vi "getRowElements.vi"(8 "error in (no error)":errorcluster, 11 "Category in":refnum<class "Category.lvclass">) -> (0 "error out":errorcluster, 2 "Row Interface":string[](array[string]), 3 "Category out":refnum<class "Category.lvclass">)   [LabVIEW 2020, in "Category.lvclass"]
uses:
  Category.lvclass
  UserEditableAmount/UserEditableAmount.lvclass
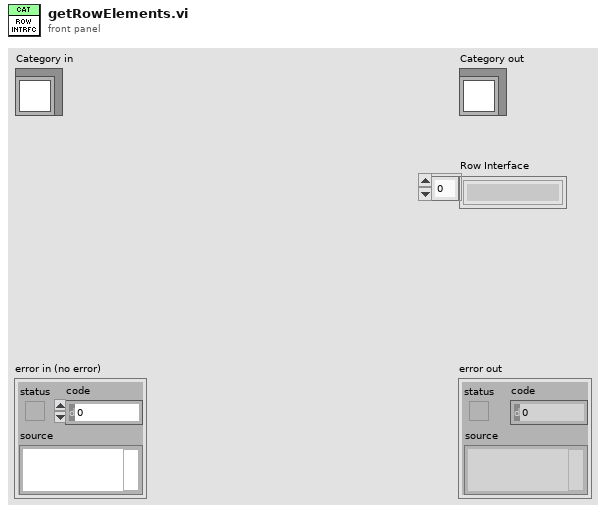
[diagram p1: front panel]
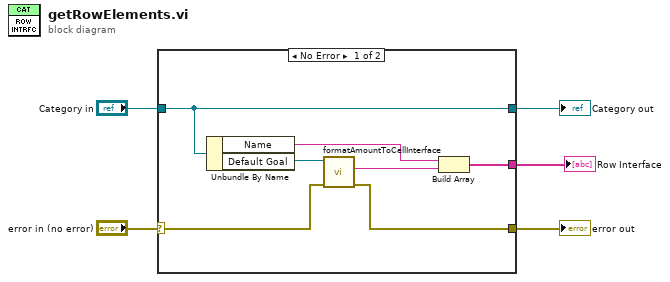
[diagram p0: block diagram]
diagram:
  n1 = case shown="No Error" "error in (no error)" {
    selector: "error in (no error)" -> [w12 w14]
    tunnel: [w11 w14] -> w4
    tunnel: [w7 w13] -> w2
    tunnel: "Category in" -> [w7 w13]
    tunnel: [w8 _] -> w1
    frame No Error {
      n2 = Unbundle By Name(w7) -> ("Name"=w10:string, "Default Goal"=w6:refnum<class "UserEditableAmount.lvclass">)
      n3 = call "formatAmountToCellInterface.vi"("error in (no error)"=w12, "UserEditableAmount in"=w6) -> ("error out"=w11:errorcluster, "Cell Interface"=w9:string)  [unwired: 7 in, 1 out]
      n4 = Build Array(w10, w9) -> (w8:string[])
    }
    frame Error {
    }
  }
  "error out" <- w4
  "Category out" <- w2
  "Row Interface" <- w1
